vi "a.vi"   [LabVIEW 2020]
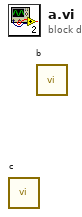
[diagram p0: block diagram]
diagram:
  n1 = call "c.vi"() -> ()  [unwired: 12 in]
  n2 = call "b.vi"() -> ()  [unwired: 12 in]
